vi "Setup Statically-Linked subWorkers.vi"(8 "error in":errorcluster, 11 "Head_ScopeSim in":refnum<class "Head_ScopeSim.lvclass">) -> (0 "error out":errorcluster, 3 "Head_ScopeSim out":refnum<class "Head_ScopeSim.lvclass">)   [LabVIEW 2019, in "Head_ScopeSim.lvclass"]
doc: "This VI performs a setup of all the statically-linked subWorkers that belong to the Worker that owns this VI. This VI must be called <b>before</b> any statically-linked subWorkers are called."
uses:
  Head_ScopeSim.lvclass
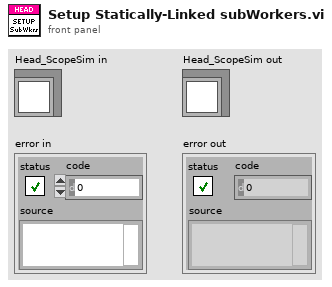
[diagram p1: front panel]
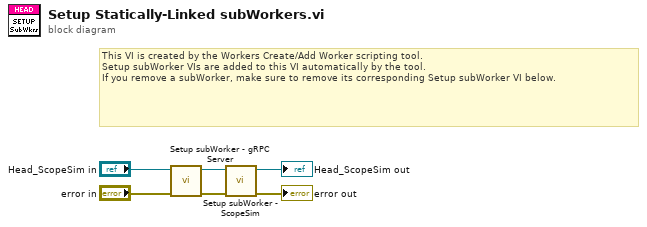
[diagram p0: block diagram]
diagram:
  # "This VI is created by the Workers Create/Add Worker scripting tool.\nSetup subWorker VIs are added to this VI automatically by the tool.\nIf you remove a subWorker, make sure to remove its corresponding Setup subWorker VI below."
  n1 = call "Setup subWorker - gRPC Server.vi"("error in"="error in", "Head_ScopeSim in"="Head_ScopeSim in") -> ("error out"=w5:errorcluster, "Head_ScopeSim out"=w2:refnum<class "Head_ScopeSim.lvclass">)  [unwired: 8 in]
  n2 = call "Setup subWorker - ScopeSim.vi"("error in"=w5, "Head_ScopeSim in"=w2) -> ("error out"=→"error out":errorcluster, "Head_ScopeSim out"=→"Head_ScopeSim out":refnum<class "Head_ScopeSim.lvclass">)  [unwired: 8 in]
